vi "Switch_Disconnect Relay.vi"(8 "error in (no error)":errorcluster, 10 "Disconnect Pins":string[](array[string]), 11 "Semiconductor Module Context":T1) -> (0 "error out":errorcluster, 3 "Semiconductor Module Context (dup)":T1)   [LabVIEW 2014]
uses:
  <vilib>/NI_TestStand_SemiconductorModule/NI_TestStand_Semiconductor_Module.lvlibp/PinMap/General/SemiconductorModuleContext.ctl
  <instrlib>/niSwitch/niSwitch.LLB/niSwitch Disconnect Channels (Single).vi
  <vilib>/NI_TestStand_SemiconductorModule/NI_TestStand_Semiconductor_Module.lvlibp
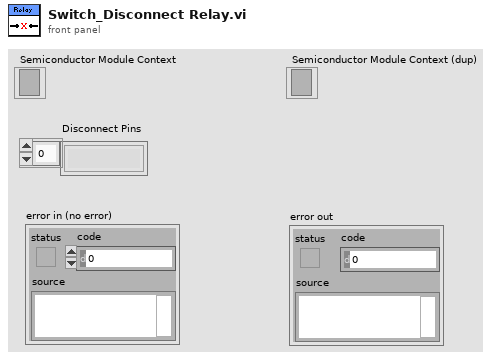
[diagram p1: front panel]
types:
  T1 = typedef "NI_TestStand_Semiconductor_Module.lvlibp/SemiconductorModuleContext.ctl" = refnum<k7>
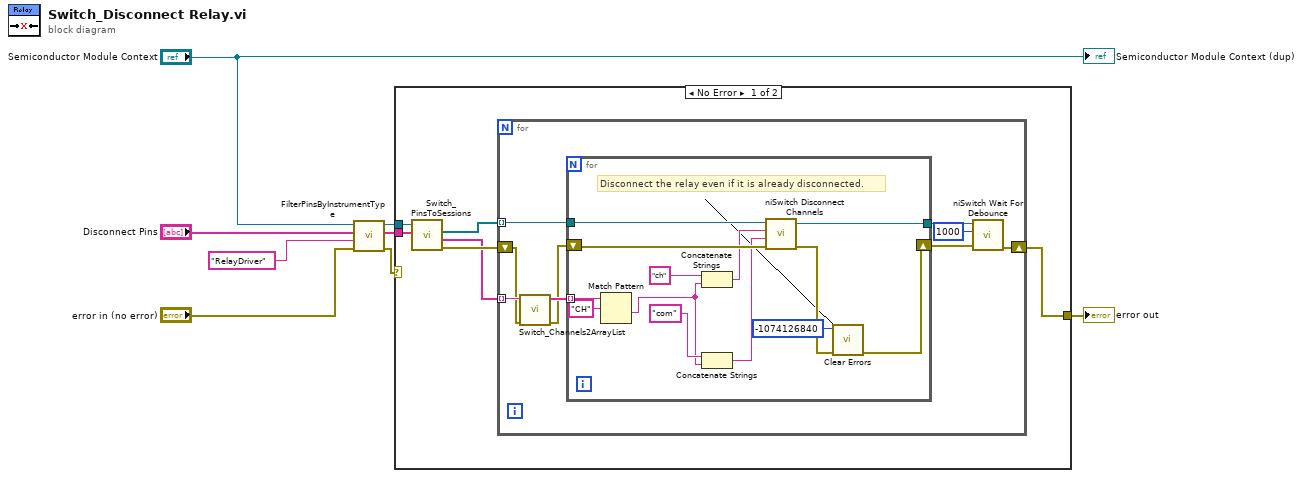
[diagram p0: block diagram]
diagram:
  n1 = call <vilib>:"FilterPinsByInstrumentType.vi"("error in (no error)"="error in (no error)", "Instrument Type Id"="RelayDriver", "Pins"="Disconnect Pins", "Semiconductor Module Context"="Semiconductor Module Context") -> ("error out"=w1:errorcluster, "Filtered Pins"=w2:string[], "Semiconductor Module Context Out"=w3:T1)  [unwired: 5 in]
  n2 = case shown="No Error" w1 {
    selector: w1 -> [_ w37]
    tunnel: [w14 w37] -> w5
    tunnel: w3 -> [w10 _]
    tunnel: w2 -> [w9 _]
    frame No Error {
      n3 = call "Switch_PinsToSessions.vi"("Pins"=w9, "Semiconductor Module Context"=w10) -> ("error out"=w13:errorcluster, "Channel Lists"=w12:string[], "Instrument Sessions"=w11:refnum<k15>[])  [unwired: 5 in, 2 out]
      n4 = for {
        shift-right: [w20] -> w14
        shift-left: w13 -> [w15]
        tunnel: w12 -> [w23] mode=indexing
        tunnel: w11 -> [w18] mode=indexing
        n5 = call "Switch_Channels2ArrayList.vi"("error in (no error)"=w15, "Channel List"=w23) -> ("error out"=w16:errorcluster, "Array of Channels"=w22:string[])  [unwired: 8 in]
        n6 = for {
          shift-right: [w25] -> w21
          shift-left: w16 -> [w36]
          tunnel: w22 -> [w28] mode=indexing
          tunnel: [w30] -> w19
          tunnel: w18 -> [w29]
          # "Disconnect the relay even if it is already disconnected."
          n7 = Match Pattern(string=w28, regular expression="CH") -> (after substring=w26:string)  [unwired: 1 in, 3 out]
          n8 = Concatenate Strings("ch" ("string"), w26) -> (w33:string)
          n9 = Concatenate Strings("com" ("string"), w26) -> (w32:string)
          n10 = call-poly <instrlib>:"niSwitch Disconnect Channels.vi"("error in (no error)"=w36, "channel 2"=w32, "channel 1"=w33, "instrument handle"=w29) -> ("error out"=w31:errorcluster, "instrument handle out"=w30:refnum<k15>)  [unwired: 6 in]
          n11 = call <vilib>:"Clear Errors.vi"("error in (no error)"=w31, "specific error code to clear (0: all)"=-1074126840) -> ("error out"=w25:errorcluster)  [unwired: 4 in, 1 out]
        }
        n12 = call <instrlib>:"niSwitch Wait For Debounce.vi"("error in (no error)"=w21, "maximum time (5000 ms)"=1000, "instrument handle"=w19) -> ("error out"=w20:errorcluster)  [unwired: 7 in, 1 out]
      }
    }
    frame Error {
    }
  }
  "error out" <- w5
  "Semiconductor Module Context (dup)" <- "Semiconductor Module Context"
